vi "Write Properties.vi"(8 "error in":errorcluster, 10 "Properties":refnum<class "Property.lvclass">[](array[class]), 11 "Item in":refnum<class "Item.lvclass">) -> (0 "error out":errorcluster, 3 "Item out":refnum<class "Item.lvclass">)   [LabVIEW 2024, in "Parser.lvlib" / "Item.lvclass"]
uses:
  Item.lvclass
  Property/Property.lvclass
  Item.lvclass/Item.ctl
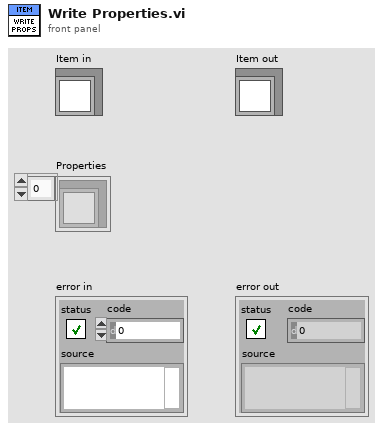
[diagram p1: front panel]
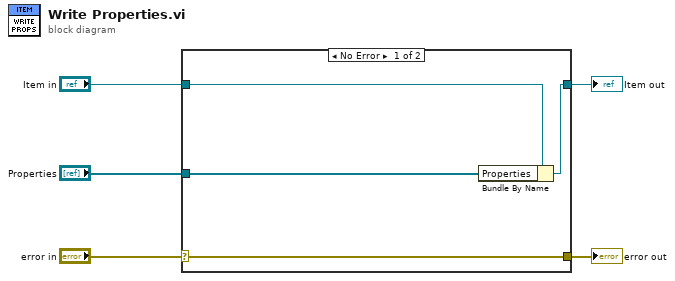
[diagram p0: block diagram]
diagram:
  n1 = case shown="No Error" "error in" {
    selector: "error in" -> [w9 w11]
    tunnel: [w9 w11] -> w4
    tunnel: [w7 w10] -> w2
    tunnel: "Item in" -> [w8 w10]
    tunnel: "Properties" -> [w6 _]
    frame No Error {
      n2 = Bundle By Name(cluster=w8, "Properties"=w6) -> (w7:refnum<class "Item.lvclass">)
    }
    frame Error {
    }
  }
  "error out" <- w4
  "Item out" <- w2
